vi "SOLSTIS_EMA_21Aug17_program.vi"(0 "Setpoint \n(MHz)":dbl=384351008.8830141 format="%#_13g", 1 "Frequency Threshold (MHz)":dbl, 2 "Change wavelength":bool, 3 "connection ID out":refnum<k5>, 4 "Bypass Check Lock":bool, 5 "error in (no error)":errorcluster) -> (6 "Actual Frequency (MHz)":dbl=384351009.3710027 format="%#_14g", 7 "Difference (MHz)":dbl=0.48798859119415283, 8 "Locked?":bool=TRUE, 9 "error out":errorcluster)   [LabVIEW 2017]
uses:
  wlmData.dll
  <vilib>/Analysis/NI_AALBase.lvlib
panel:
  out "start time (ms)":u32
  in  "?":bool
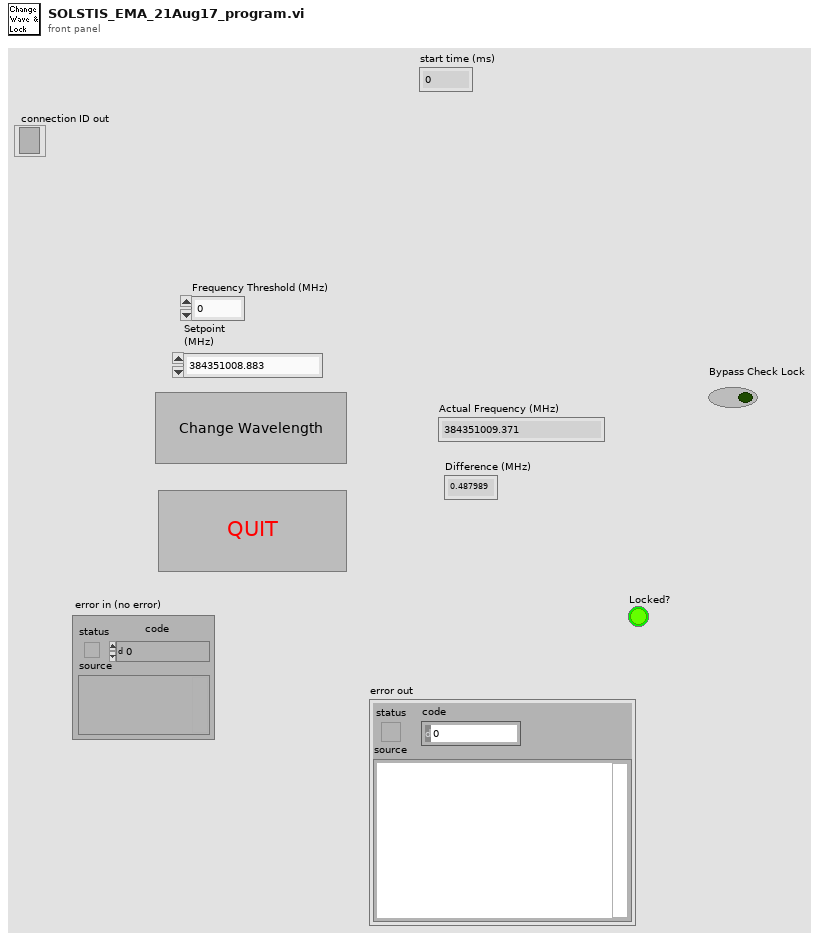
[diagram p1: front panel]
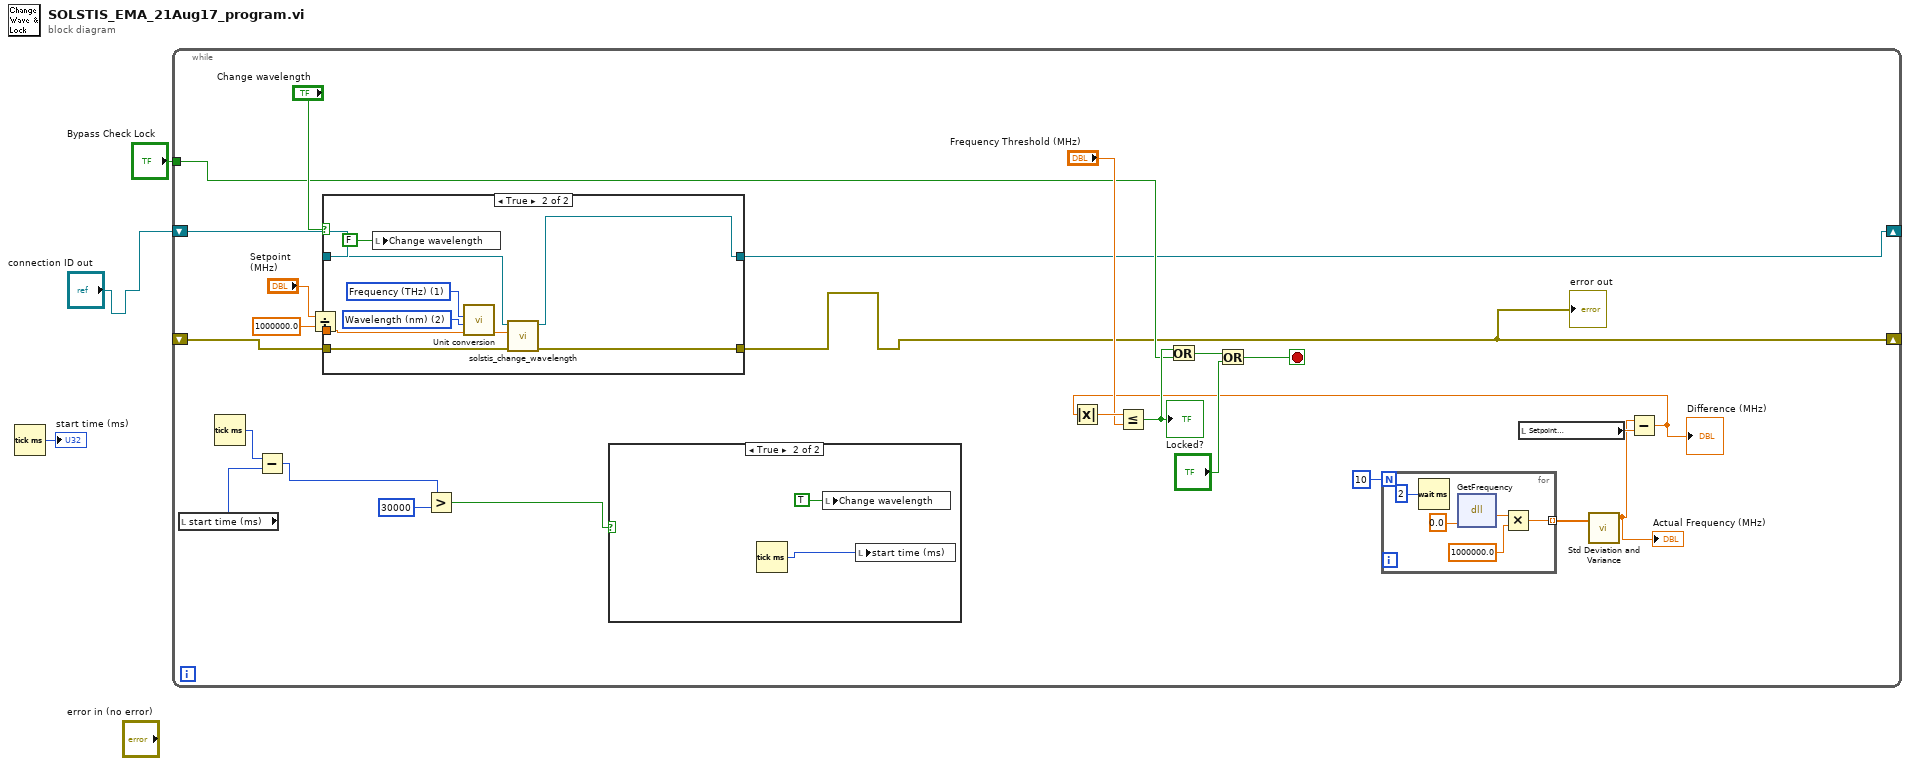
[diagram p0: block diagram]
diagram:
  n1 = Tick Count (ms)() -> (millisecond timer value=→"start time (ms)":u32)
  n2 = while {
    shift-right: [w18] -> _
    shift-left: "connection ID out" -> [w27]
    shift-right: [w4] -> _
    shift-left: _ -> [w26]
    tunnel: "Bypass Check Lock" -> [w19]
    stop <- w22 stop-if-true
    n3 = local read "start time (ms)"() -> (w6:u32)
    n4 = Tick Count (ms)() -> (millisecond timer value=w7:u32)
    n5 = Subtract(x=w7, y=w6) -> (x-y=w5:u32)
    n6 = Divide(x="Setpoint \n(MHz)", y=1000000.0) -> (x/y=w16:dbl)
    n7 = case shown="True" "Change wavelength" {
      tunnel: w27 -> [w37 w45]
      tunnel: [w37 w42] -> w18
      tunnel: w26 -> [w36 w44]
      tunnel: [w36 w43] -> w4
      tunnel: w16 -> [_ w39]
      frame False {
      }
      frame True {
        w40 = u16 2 items=["Wavenumber (cm-1)", "Frequency (THz)", "Wavelength (nm)"] ("Ending Units")
        w41 = u16 1 items=["Wavenumber (cm-1)", "Frequency (THz)", "Wavelength (nm)"] ("Starting Units")
        n8 = local write "Change wavelength"(FALSE) -> ()
        n9 = call "Unit conversion.vi"("Value to convert"=w39, "Ending Units"=w40, "Starting Units"=w41) -> ("Output"=w38:dbl)  [unwired: 8 out]
        n10 = call "solstis_change_wavelength.vi"("error in (no error)"=w44, "Setpoint(nm)"=w38, "connection ID"=w45) -> ("error out"=w43:errorcluster, "connection ID out"=w42:refnum<k5>)  [unwired: 7 out]
      }
    }
    "error out" <- w4
    n11 = Greater?(x=w5, y=u32 30000) -> (0:w8:bool)
    n12 = case shown="True" w8 {
      frame False {
      }
      frame True {
        n13 = Tick Count (ms)() -> (millisecond timer value=w29:u32)
        n14 = local write "Change wavelength"(TRUE ("Change wavelength")) -> ()
        n15 = local write "start time (ms)"(w29) -> ()
      }
    }
    n16 = for {
      N: 10 -> [_]
      tunnel: [w32] -> w13 mode=indexing
      n17 = Wait (ms)(milliseconds to wait=u32 2) -> ()  [unwired: 1 out]
      n18 = dll-call lib="wlmData.dll" fn="GetFrequency"("arg1"=0.0) -> ("return type"=w34:dbl)  [unwired: 4 in, 2 out]
      n19 = Multiply(x=w34, y=1000000.0) -> (x*y=w32:dbl)
    }
    n20 = local read "Setpoint \n(MHz)"() -> (w12:dbl)
    n21 = call <vilib>:"Std Deviation and Variance.vi"("X"=w13) -> ("mean"=w11:dbl)  [unwired: 1 in, 2 out]
    "Actual Frequency (MHz)" <- w11
    n22 = Subtract(x=w11, y=w12) -> (x-y=w10:dbl)
    "Difference (MHz)" <- w10
    n23 = Absolute Value(x=w10) -> (abs(x)=w24:dbl)
    n24 = Less Or Equal?(x=w24, y="Frequency Threshold (MHz)") -> (x <= y?=w21:bool)
    "Locked?" <- w21
    n25 = Or(x=w21, y=w19) -> (x .or. y?=w20:bool)
    n26 = Or(x=w20, y="?") -> (x .or. y?=w22:bool)
  }
